vi "Simula stato PLC_2.vi"(11 "USCITE PLC":T1) -> (3 "STATO PLC":T4)   [LabVIEW 2019]
uses:
  STATO PLC 2.ctl
  Uscite PLC 2.ctl
  controls/statoAO_plc_2.ctl
  StatoDO_PLC_2.ctl
panel:
  in  "Stato DI_PLC.Reset da pulsantiera":bool
  in  "Stato DI_PLC.Stop da pulsantiera":bool
  in  "Stato DI_PLC.Start da pulsantiera":bool
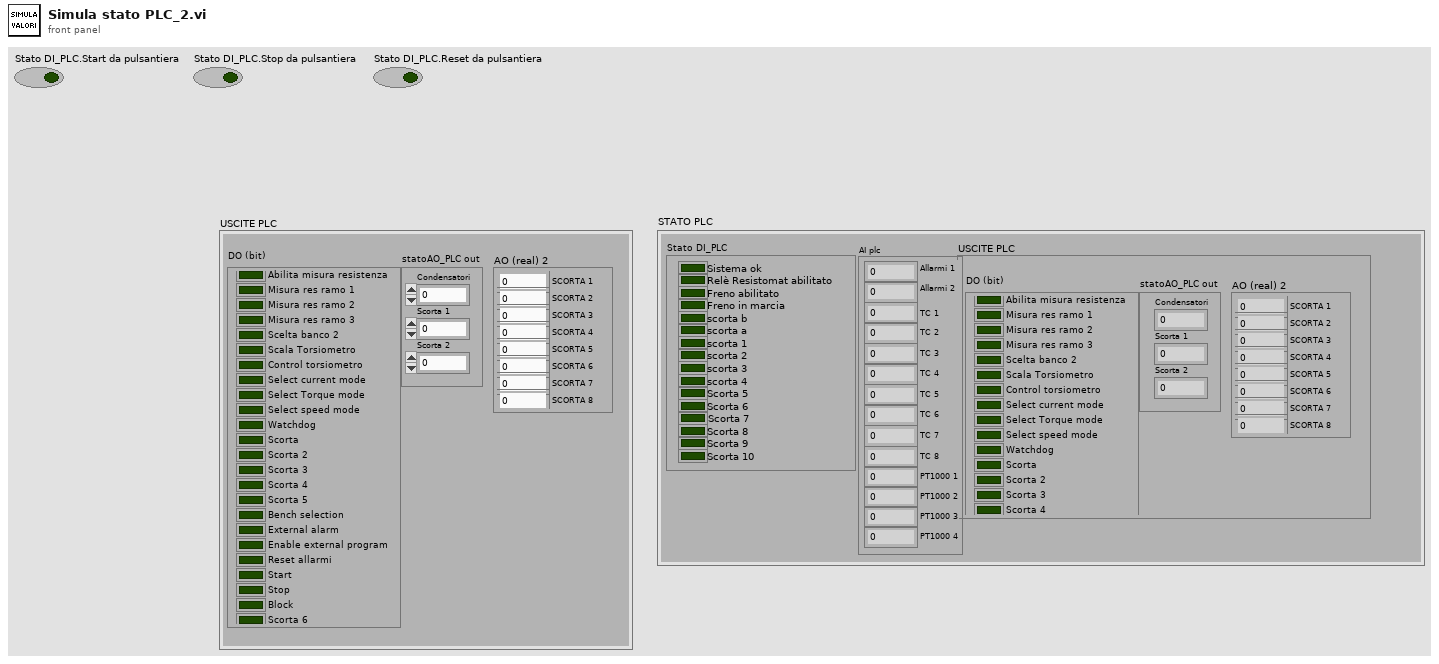
[diagram p1: front panel]
types:
  T1 = typedef "Uscite PLC 2.ctl" = cluster{"AO (real) 2":cluster{"SCORTA 1":dbl, "SCORTA 2":dbl, "SCORTA 3":dbl, "SCORTA 4":dbl, "SCORTA 5":dbl, "SCORTA 6":dbl, "SCORTA 7":dbl, "SCORTA 8":dbl}, "statoAO_PLC out":T2, "DO (bit)":T3}
  T2 = typedef "statoAO_plc_2.ctl" = cluster{"Condensatori":dbl, "Scorta 1":dbl, "Scorta 2":dbl}
  T3 = typedef "StatoDO_PLC_2.ctl" = cluster{"Relè misura resistomat":bool, "Misura res ramo 1":bool, "Misura res ramo 2":bool, "Misura res ramo 3":bool, "Scelta banco 2":bool, "Scala Torsiometro":bool, "Ctrl torsiometro":bool, "Select current mode":bool, "Select Torque mode":bool, "Select speed mode":bool, "Watchdog":bool, "Scorta":bool, "Scorta 2":bool, "Scorta 3":bool, "Scorta 4":bool, "Scorta 5":bool, "Bench selection":bool, "External alarm":bool, "Enable external program":bool, "Reset allarmi":bool, "Start":bool, "Stop":bool, "Block":bool, "Scorta 6":bool}
  T4 = typedef "STATO PLC 2.ctl" = cluster{"USCITE PLC":T1, "Stato DI_PLC":cluster{"Sistema ok":bool, "Relè Resistomat abilitato":bool, "Freno abilitato":bool, "Freno in marcia":bool, "scorta b":bool, "scorta a":bool, "scorta 1":bool, "scorta 2":bool, "scorta 3":bool, "scorta 4":bool, "Scorta 5":bool, "Scorta 6":bool, "Scorta 7":bool, "Scorta 8":bool, "Scorta 9":bool, "Scorta 10":bool}, "AI plc":cluster{"Allarmi 1":dbl, "Allarmi 2":dbl, "TC 1":dbl, "TC 2":dbl, "TC 3":dbl, "TC 4":dbl, "TC 5":dbl, "TC 6":dbl, "TC 7":dbl, "TC 8":dbl, "PT1000 1":dbl, "PT1000 2":dbl, "PT1000 3":dbl, "PT1000 4":dbl}}
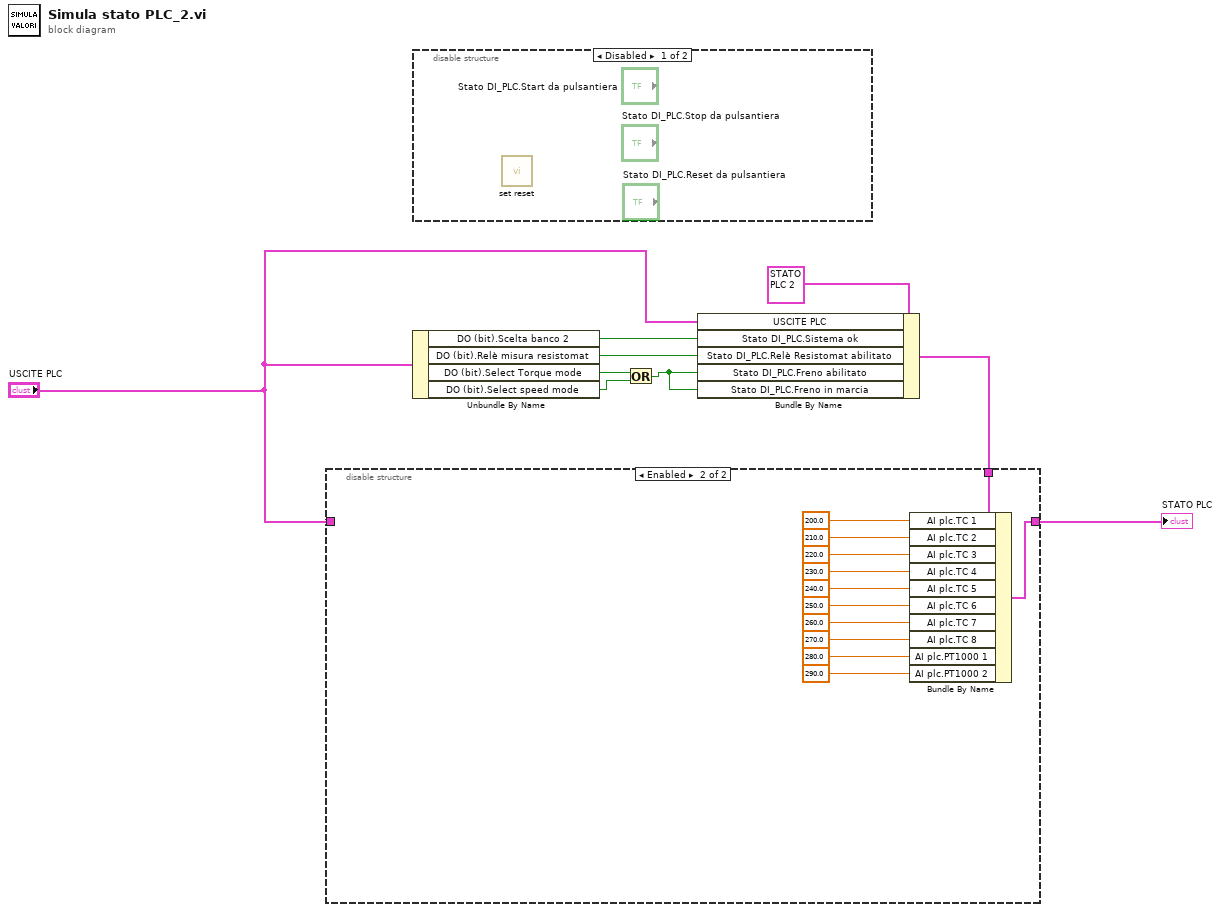
[diagram p0: block diagram]
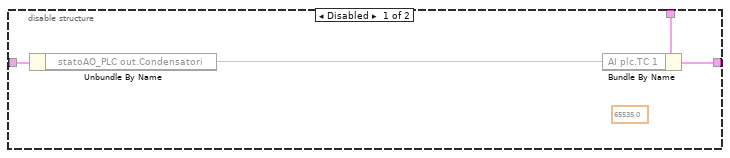
[diagram p2: hidden frame]
diagram:
  n1 = Unbundle By Name("USCITE PLC") -> ("DO (bit).Scelta banco 2"=w4:bool, "DO (bit).Relè misura resistomat"=w5:bool, "DO (bit).Select Torque mode"=w3:bool, "DO (bit).Select speed mode"=w2:bool)
  n2 = disable-structure shown="Disabled" {
    frame Disabled {
      n3 = call "set reset.vi"() -> ()  [unwired: 11 in, 1 out]
    }
    frame Enabled {
    }
  }
  n4 = Or(x=w3, y=w2) -> (x .or. y?=w1:bool)
  n5 = Bundle By Name(cluster=T4 {"USCITE PLC"={"AO (real) 2"={"SCORTA 1"=0.0, "SCORTA 2"=0.0, "SCORTA 3"=0.0, "SCORTA 4"=0.0, "SCORTA 5"=0.0, "SCORTA 6"=0.0, "SCORTA 7"=0.0, "SCORTA 8"=0.0}, "statoAO_PLC out"={"Condensatori"=0.0, "Scorta 1"=0.0, "Scorta 2"=0.0}, "DO (bit)"={"Relè misura resistomat"=FALSE, "Misura res ramo 1"=FALSE, "Misura res ramo 2"=FALSE, "Misura res ramo 3"=FALSE, "Scelta banco 2"=FALSE, "Scala Torsiometro"=FALSE, "Ctrl torsiometro"=FALSE, "Select current mode"=FALSE, "Select Torque mode"=FALSE, "Select speed mode"=FALSE, "Watchdog"=FALSE, "Scorta"=FALSE, "Scorta 2"=FALSE, "Scorta 3"=FALSE, "Scorta 4"=FALSE, "Scorta 5"=FALSE, "Bench selection"=FALSE, "External alarm"=FALSE, "Enable external program"=FALSE, "Reset allarmi"=FALSE, "Start"=FALSE, "Stop"=FALSE, "Block"=FALSE, "Scorta 6"=FALSE}}, "Stato DI_PLC"={"Sistema ok"=FALSE, "Relè Resistomat abilitato"=FALSE, "Freno abilitato"=FALSE, "Freno in marcia"=FALSE, "scorta b"=FALSE, "scorta a"=FALSE, "scorta 1"=FALSE, "scorta 2"=FALSE, "scorta 3"=FALSE, "scorta 4"=FALSE, "Scorta 5"=FALSE, "Scorta 6"=FALSE, "Scorta 7"=FALSE, "Scorta 8"=FALSE, "Scorta 9"=FALSE, "Scorta 10"=FALSE}, "AI plc"={"Allarmi 1"=0.0, "Allarmi 2"=0.0, "TC 1"=0.0, "TC 2"=0.0, "TC 3"=0.0, "TC 4"=0.0, "TC 5"=0.0, "TC 6"=0.0, "TC 7"=0.0, "TC 8"=0.0, "PT1000 1"=0.0, "PT1000 2"=0.0, "PT1000 3"=0.0, "PT1000 4"=0.0}} ("STATO PLC"), "USCITE PLC"="USCITE PLC", "Stato DI_PLC.Sistema ok"=w4, "Stato DI_PLC.Relè Resistomat abilitato"=w5, "Stato DI_PLC.Freno abilitato"=w1, "Stato DI_PLC.Freno in marcia"=w1) -> (w9:T4)
  n6 = disable-structure shown="Enabled" {
    disable-tunnel: w9 -> [w13 w25]
    disable-tunnel: [w12 w24] -> w8
    disable-tunnel: "USCITE PLC" -> [w10 _]
    frame Disabled {
      (unwired) 65535.0 ("AI plc.Allarmi")
      n7 = Unbundle By Name(w10) -> ("statoAO_PLC out.Condensatori"=w11:dbl)
      n8 = Bundle By Name(cluster=w13, "AI plc.TC 1"=w11) -> (w12:T4)
    }
    frame Enabled {
      n9 = Bundle By Name(cluster=w25, "AI plc.TC 1"=200.0, "AI plc.TC 2"=210.0 ("AI plc.TC 1"), "AI plc.TC 3"=220.0 ("AI plc.TC 1"), "AI plc.TC 4"=230.0 ("AI plc.TC 1"), "AI plc.TC 5"=240.0 ("AI plc.TC 1"), "AI plc.TC 6"=250.0 ("AI plc.TC 1"), "AI plc.TC 7"=260.0 ("AI plc.TC 1"), "AI plc.TC 8"=270.0 ("AI plc.TC 1"), "AI plc.PT1000 1"=280.0 ("AI plc.TC 1"), "AI plc.PT1000 2"=290.0 ("AI plc.TC 1")) -> (w24:T4)
    }
  }
  "STATO PLC" <- w8
